vi "Intake Reach Height.vi"(5 "PID gains":T1={"proportional gain (Kc)"=1.0, "integral time (Ti, min)"=0.01, "derivative time (Td, min)"=0.0} {"derivative time (Td, min)" format="%.3f"; "integral time (Ti, min)" format="%.3f"; "proportional gain (Kc)" format="%.3f"}, 7 "output range":cluster{"output high":dbl, "output low":dbl}={"output high"=100.0, "output low"=-100.0} {"output low" format="%.2f"; "output high" format="%.2f"}, 9 "Reach Height":dbl, 10 "Current Height":dbl format="%.2f", 11 "Tolerance":dbl) -> (1 "Finished":bool, 2 "Output":dbl)   [LabVIEW 2017]
uses:
  Common Code/PID Gains.ctl
  <vilib>/addons/control/pid/pid.llb/PID (DBL).vi
  <vilib>/addons/control/pid/NI_PID_pid.lvlib
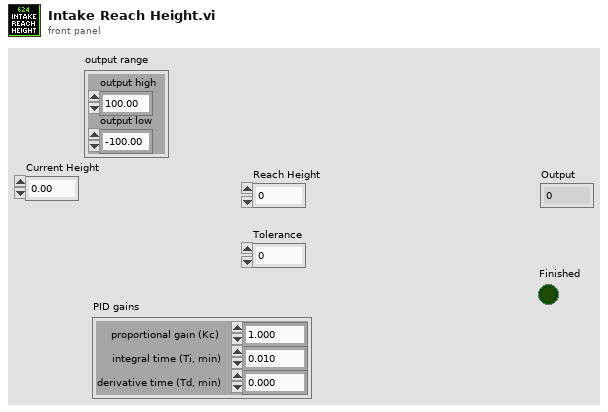
[diagram p1: front panel]
types:
  T1 = typedef "PID Gains.ctl" = cluster{"proportional gain (Kc)":dbl, "integral time (Ti, min)":dbl, "derivative time (Td, min)":dbl}
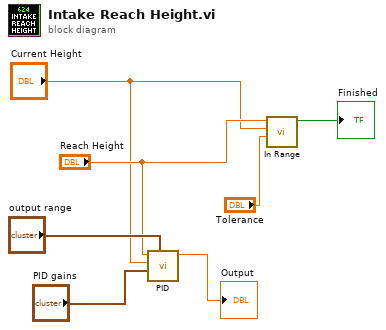
[diagram p0: block diagram]
diagram:
  n1 = call-poly <vilib>:"PID.vi"("output range"="output range", "PID gains"="PID gains", "process variable"="Current Height", "setpoint"="Reach Height") -> ("output"=→"Output":dbl)  [unwired: 6 in, 1 out]
  n2 = call "In Range.vi"("Tolerance"="Tolerance", "Encoder Height"="Current Height", "Height"="Reach Height") -> ("In Range"=→"Finished":bool)  [unwired: 8 in]
